vi "String Contains.vi"(11 "Data In":string) -> (3 "Data Out":string)   [LabVIEW 2016]
uses:
  Core/Assert API Components/Failure Actions.ctl
  Core/Assert API Components/VI References.ctl
  Core/Assert API Components/Assert API Components.lvlib
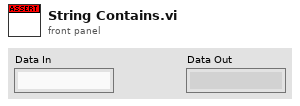
[diagram p1: front panel]
types:
  T1 = typedef "Assert API Components.lvlib/VI References.ctl" = cluster{"Calling VI Ref":refnum<vi>, "Assert VI Ref":refnum<vi>}
  T2 = typedef "Assert API Components.lvlib/Failure Actions.ctl" = enum16{"None", "Log To File", "Pause Execution", "Abort Execution"}
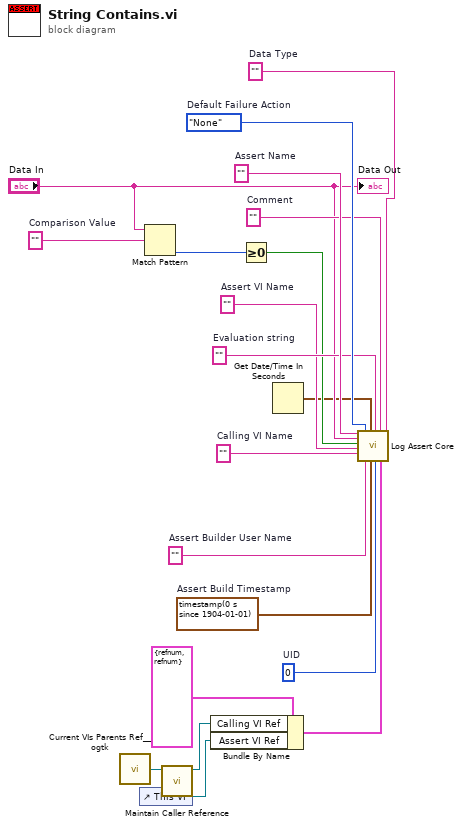
[diagram p0: block diagram]
diagram:
  w3 = 0  # UID
  w4 = ""  # Assert VI Name
  w5 = ""  # Calling VI Name
  w6 = timestamp(0 s since 1904-01-01)  # Assert Build Timestamp
  w7 = ""  # Assert Builder User Name
  w8 = ""  # Data Type
  w18 = ""  # Comment
  w17 = ""  # Evaluation string
  w19 = Failure_Actions."None"  # Default Failure Action
  w20 = ""  # Assert Name
  w15 = ""  # Comparison Value
  n1 = call <userlib>:"Current VIs Parents Ref__ogtk.vi"() -> ("Calling VI's Reference"=w11:refnum<vi>)  [unwired: 2 in]
  n2 = control-ref of="This VI"() -> (w10:refnum<vi>)
  n3 = Match Pattern(string="Data In", regular expression=w15) -> (offset past match=w14:i32)  [unwired: 1 in, 3 out]
  n4 = call "Maintain Caller Reference.vi"("VI in"=w11) -> ("VI out"=w2:refnum<vi>)  [unwired: 10 in]
  n5 = Bundle By Name(cluster=T1 {"Calling VI Ref"=refnum, "Assert VI Ref"=refnum} ("VI References"), "Calling VI Ref"=w2, "Assert VI Ref"=w10) -> (w9:T1)
  n6 = Greater Or Equal To 0?(x=w14) -> (x >= 0?=w13:bool)
  n7 = Get Date/Time In Seconds() -> (seconds since 1Jan1904=w1:timestamp)
  n8 = call "Log Assert Core.vi"("Assert Name"=w20, "Data Value"="Data In", "Status"=w13, "Assert VI Name"=w4, "Calling VI Name"=w5, "Failure Action"=w19, "Assert Builder User Name"=w7, "Last Update"=w1, "Assert Build Timestamp"=w6, "Evaluation String"=w17, "Assert VI UID"=w3, "Comment"=w18, "VI References"=w9, "Data Type"=w8) -> ()  [unwired: 6 in]
  "Data Out" <- "Data In"
